vi "AC2250 Measure (Main).vi"(8 "ErrIn":errorcluster, 11 "VISA Resource Name In":refnum<visa-resource-name>) -> (0 "ErrOut":errorcluster, 2 "Value":dbl format="%.3f", 3 "VISA Resource Name Out":refnum<visa-resource-name>, 4 "Num Chars":i32, 5 "String Received":string)   [LabVIEW 2013]
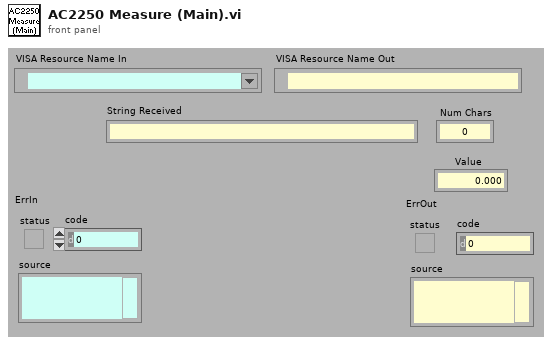
[diagram p1: front panel]
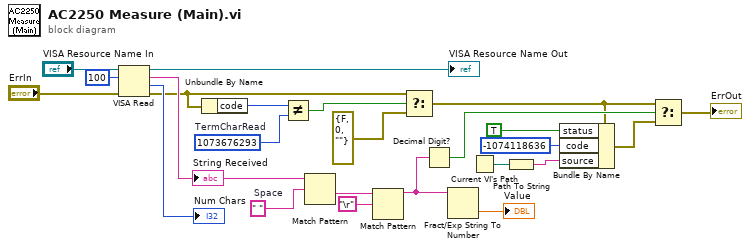
[diagram p0: block diagram]
diagram:
  w13 = 1073676293  # TermCharRead
  w18 = " "  # Space
  n1 = VISA Read(VISA resource name="VISA Resource Name In", byte count=u32 100, error in (no error)="ErrIn") -> (VISA resource name out=→"VISA Resource Name Out":refnum<visa-resource-name>, read buffer=w19:string, return count=→"Num Chars":u32, error out=w11:errorcluster)
  "String Received" <- w19
  n2 = Unbundle By Name(w11) -> ("code"=w14:i32)
  n3 = Not Equal?(x=w14, y=w13) -> (x != y?=w12:bool)
  n4 = Match Pattern(string=w19, regular expression=w18) -> (after substring=w17:string)  [unwired: 1 in, 3 out]
  n5 = Match Pattern(string=w17, regular expression="\r") -> (before substring=w9:string)  [unwired: 1 in, 3 out]
  n6 = Select(t=w11, s=w12, f=errorcluster {"status"=FALSE, "code"=0, "source"=""} ("ErrOut")) -> (s? t:f=w7:errorcluster)
  n7 = Decimal Digit?(1:w9) -> (0:w8:bool)
  n8 = Fract/Exp String To Number(string=w9) -> (number=→"Value":dbl)  [unwired: 3 in, 1 out]
  n9 = Current VI's Path() -> (path=w4:path)
  n10 = Path To String(path=w4) -> (string=w3:string)
  n11 = Bundle By Name(cluster=w7, "status"=TRUE, "code"=-1074118636, "source"=w3) -> (w2:errorcluster)
  n12 = Select(t=w7, s=w8, f=w2) -> (s? t:f=→"ErrOut":errorcluster)
